vi "Average.vi"(10 "Digitizer Samples":dbl[](array[numeric])) -> (1 "VRECT Ripple (pk-pk)":dbl, 2 "VRECT":dbl format="%0.2f")   [LabVIEW 2010]
uses:
  <vilib>/Analysis/NI_AALBase.lvlib
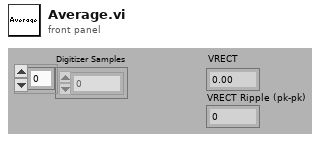
[diagram p1: front panel]
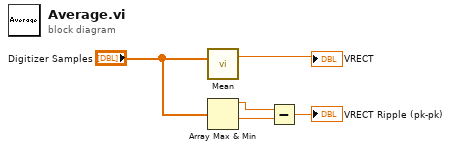
[diagram p0: block diagram]
diagram:
  n1 = call <vilib>:"Mean.vi"("X"="Digitizer Samples") -> ("mean"=→"VRECT":dbl)  [unwired: 1 out]
  n2 = Array Max & Min(array="Digitizer Samples") -> (max value=w4:dbl, min value=w3:dbl)  [unwired: 2 out]
  n3 = Subtract(x=w4, y=w3) -> (x-y=→"VRECT Ripple (pk-pk)":dbl)
